vi "Mode Est Acquire Data (TEMP).vi"(7 "Simulation Method":T3(ring), 8 "Simulation?":bool) -> ()   [LabVIEW 2017]
uses:
  <vilib>/Analysis/NI_AALPro.lvlib
  <vilib>/Analysis/NI_AALBase.lvlib
  <vilib>/addons/Control Design/_Time Response Analysis/NI_CD_Time Response.lvlib
  <vilib>/addons/Control Design/_Time Response Analysis/Time Response.llb/Time Response subVI/cd_Linear Simulation (Transfer Function).vi
  <vilib>/addons/Control Design/_Dynamic Analysis/NI_CD_Dynamic Analysis.lvlib
  <vilib>/addons/Control Design/_Dynamic Analysis/Dynamic Analysis.llb/Dynamic Analysis subVI/cd_Damping Ratio and Natural Frequency (Transfer Function).vi
  <vilib>/addons/Control Design/_Model Construction/NI_LinSys_Model Creation.lvlib
  <vilib>/addons/Control Design/_Model Construction/Model Creation.llb/Model Creation SubVI/cd_Create Transfer Function Model.vi
  <vilib>/addons/Control Design/_Model Construction/NI_LinSys_Model Information.lvlib
  <vilib>/addons/Control Design/_Model Construction/Model Information.llb/Model Information SubVIs/cd_Set Names To TF Model.vi
  <vilib>/addons/Control Design/_Utility/NI_CD_Model Viewer.lvlib
  <vilib>/addons/Control Design/_Utility/Model Viewer.llb/Model Viewer SubVI/cd_Draw Transfer Function Equation (TF).vi
  <vilib>/imath/engines/lvmath2/RunTimeEngine/Managers/WorkSpace/UID Generator.vi
  <vilib>/imath/engines/lvmath2/RunTimeEngine/ErrorHandling/NIMS_Error From Error Code.vi
  <vilib>/imath/engines/lvmath2/RunTimeEngine/LocalVariableDefStatement/MC_LocalVariableDefStatement_Display.vi
  <vilib>/imath/engines/lvmath2/RunTimeEngine/RunTimeType/NIMS_RunTimeType_From StrictType (excl LVString).vi
  <vilib>/imath/engines/lvmath2/RunTimeEngine/Managers/SymbolTable/Clear UID.vi
  <vilib>/imath/engines/lvmath2/RunTimeEngine/Managers/SymbolTable/NIMS_WorkSpace.lvlib
  <vilib>/imath/engines/lvmath2/RunTimeEngine/NodeEndStatement/NIMS_NodeEndStatement_Output.vi
  <vilib>/imath/engines/lvmath2/RunTimeEngine/ErrorHandling/NIMS_Finalize Error.vi
  <vilib>/imath/engines/lvmath2/RunTimeEngine/BuiltInFunctions/zpk_to_tf/NIMS_zpk_to_tf.vi
  <vilib>/imath/engines/lvmath/Plug In/_Char/NIMS_CH_String to Character Array.vi
  <vilib>/imath/engines/lvmath2/RunTimeEngine/BuiltInFunctions/fread_csv/NIMS_fread_csv(Str,I32,I32).vi
  <vilib>/imath/engines/lvmath/Plug In/_Char/NIMS_CH_Character RV to String.vi
  sources/support/libs/PMU Buffer/Buffer DATA OUT ordered.ctl
  sources/support/libs/PMU Buffer/PMU data buffer.lvlib
panel:
  in  "Signal Selection":T1(radio)=enum."Analog"
  in  "Sampling Frequency (Hz)":dbl=50.0
  out "Waveform out":waveform(dbl)
  in  "Output":T2
  in  "Acquisition Settings":enum32{"Test", "Simulation", "Options"}(tab)
  in  "Input Poles":cdb[](array[numeric])
  in  "Input Zeros":cdb[](array[numeric])
  in  "CSV File Input (Coefficients)":string
  out "Input Transfer Function":picture
  in  "Input Frequency (Hz)":dbl
  in  "Input Damping Ratio (%)":dbl
  out "Natural Frequencies":dbl[](array[numeric]) format="%.2f"
  out "Damping Ratios (%)":dbl[](array[numeric]) format="%.2f"
  out "Poles":cdb[](array[numeric]) format="%.2f"
  out "Simulation":bool
  # "Create Cluster for simulation inputs"
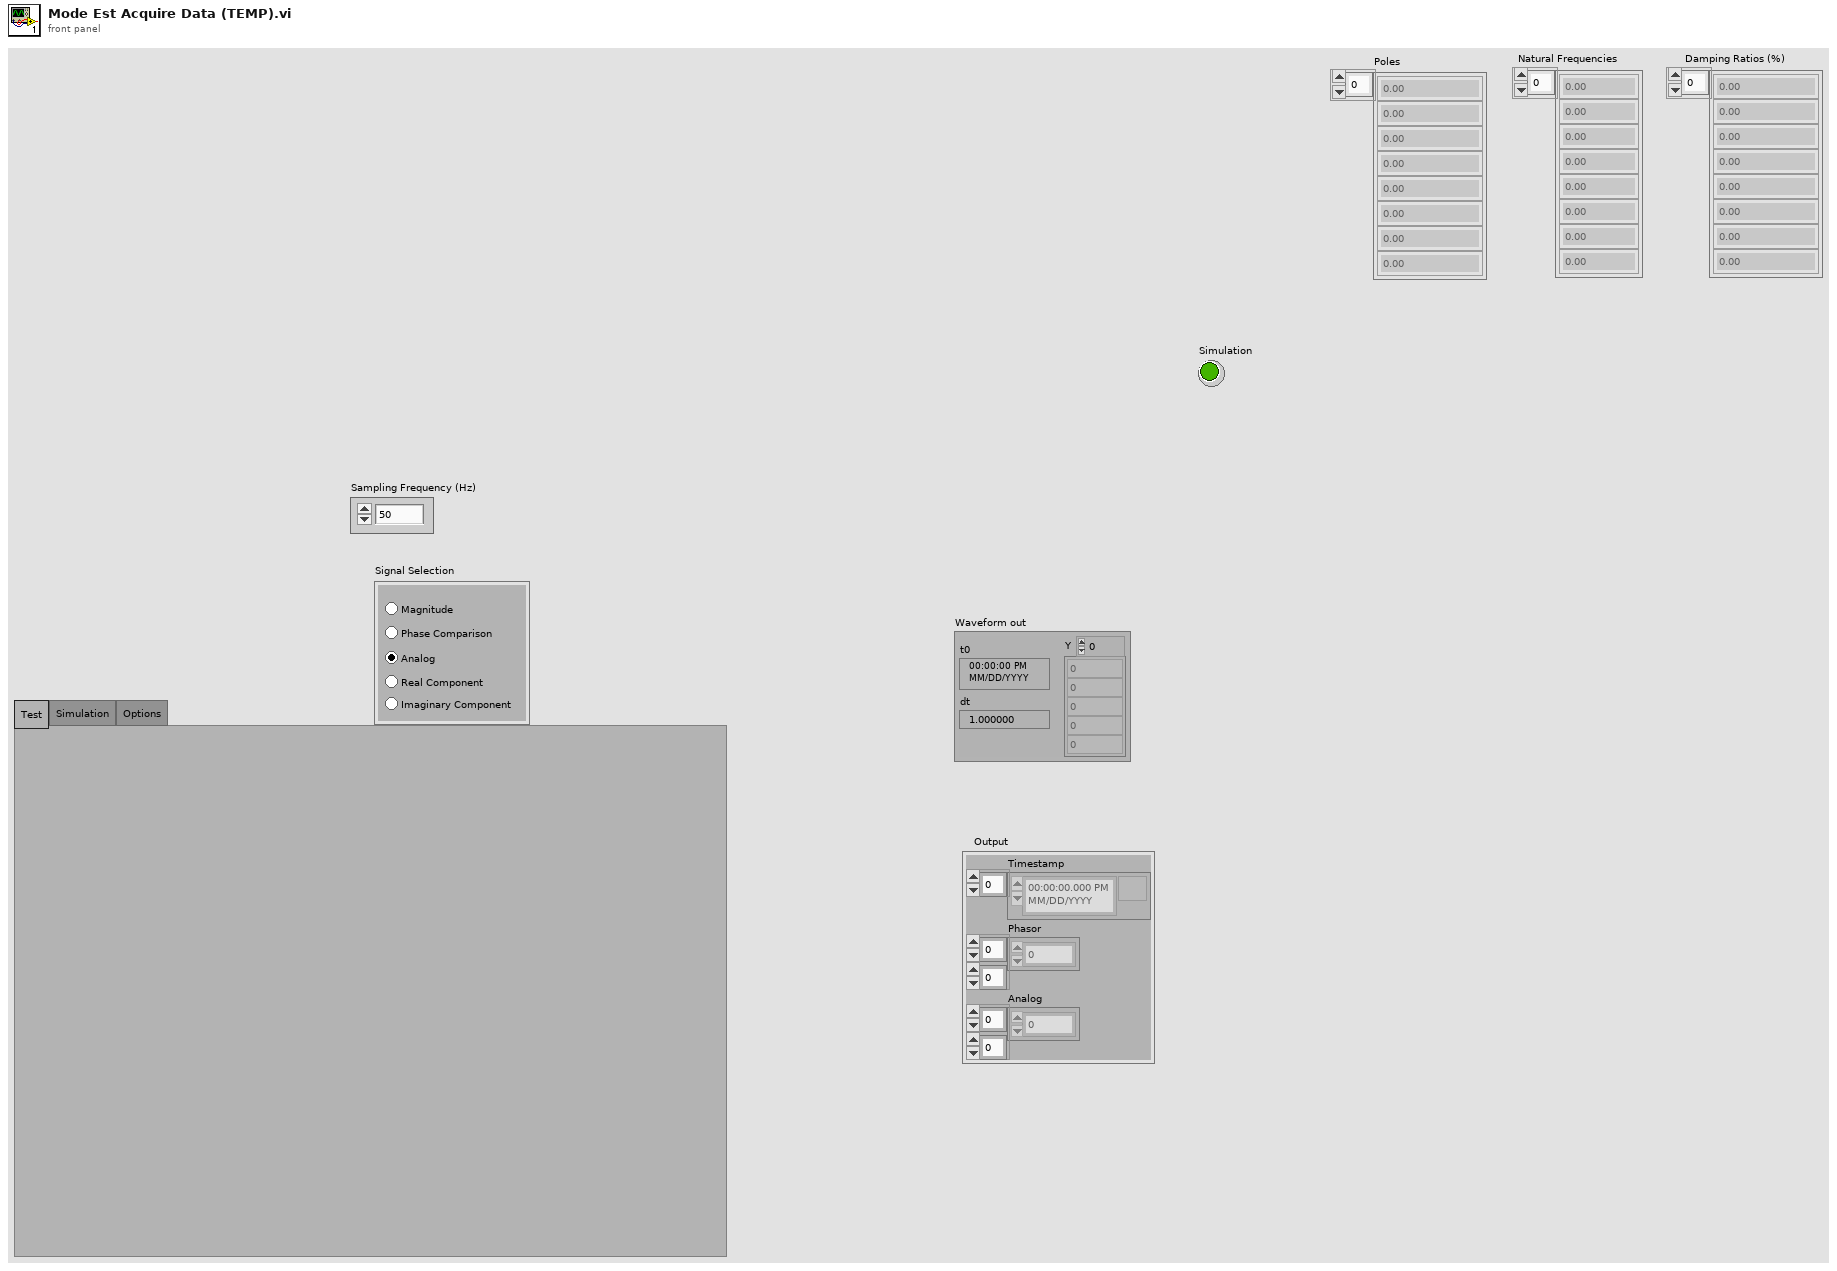
[diagram p1: front panel]
types:
  T1 = enum32{"Mag", "Phase Comparison", "Analog", "Real Component", "Imaginary Component"}
  T2 = typedef "PMU data buffer.lvlib/Buffer DATA OUT ordered.ctl" = cluster{"Timestamp":timestamp[], "Phasor":csg[][], "Analog":sgl[][]}
  T3 = enum16{"Read Coefficients (CSV)", "Use Input Frequency/D.R.", "Use Input Poles/Zeroes"}
  T4 = typedef "NI_LinSys_Model Typedefs.lvlib/CD Transfer Function Model (MIMO).ctl" = cluster{"properties":T5, "transfer function(s)":T6[][]}
  T5 = typedef "NI_LinSys_Model Typedefs.lvlib/CD General Elements.ctl" = cluster{"Model name":string, "Input names":string[], "Output names":string[], "Input Delays":dbl[], "Output Delays":dbl[], "Sampling Time":dbl, "Notes":string}
  T6 = typedef "NI_LinSys_Model Typedefs.lvlib/CD Transfer Function Model (SISO).ctl" = cluster{"Numerator":dbl[], "Denominator":dbl[], "delay":dbl}
  T7 = typedef "NI_LinSys_Data Typedefs.lvlib/CD MIMO Time Response Data.ctl" = cluster{"Time":dbl[], "Outputs Data":dbl[][][], "States Data":dbl[][][], "plot type":T8}
  T8 = typedef "NI_LinSys_Data Typedefs.lvlib/CD Plot Types Enum.ctl" = enum16{"bode-magnitude", "bode-phase", "nichols", "nyquist", "singular values", "step", "impulse", "initial", "simulation", "nyquist with separation"}
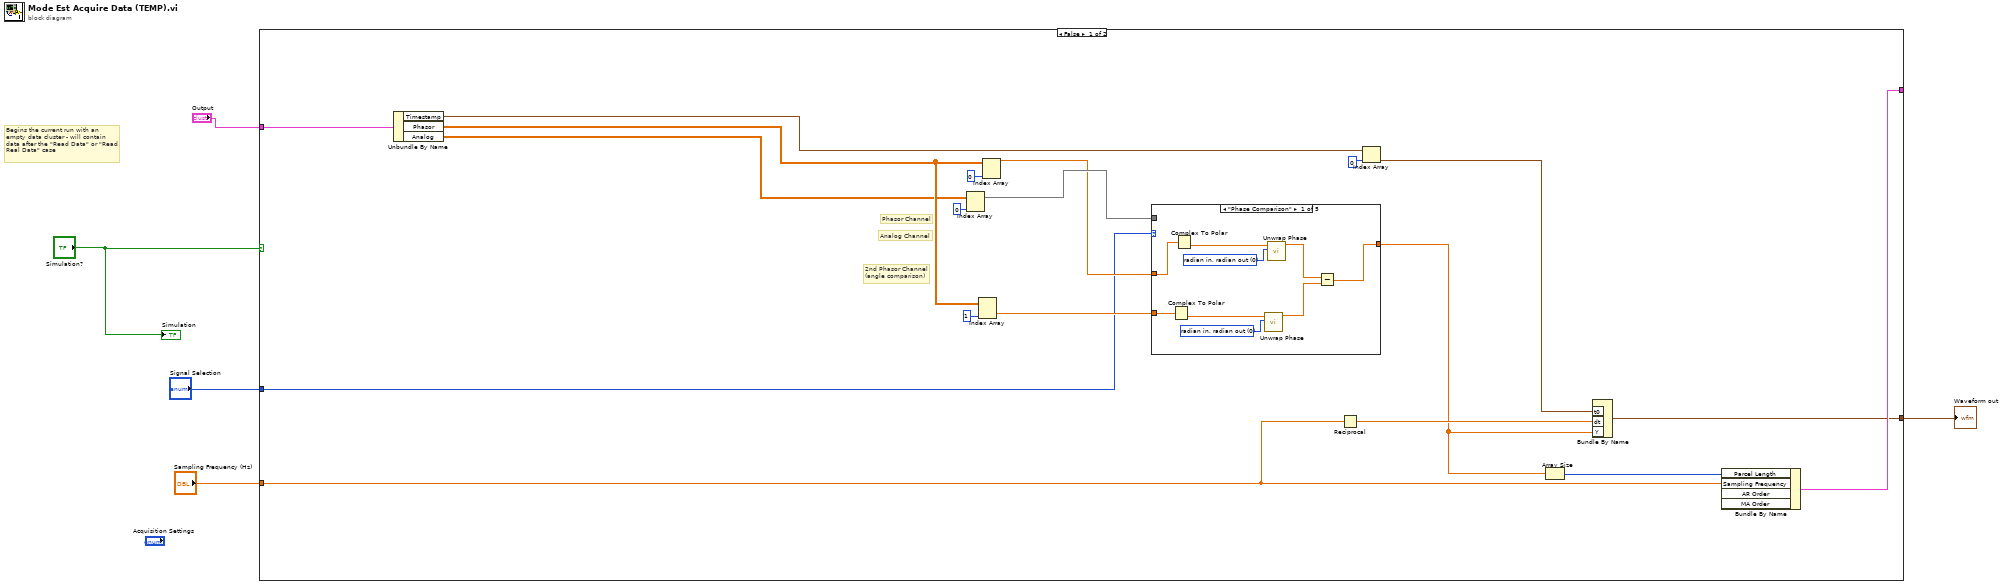
[diagram p0: block diagram]
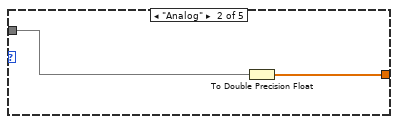
[diagram p2: hidden frame]
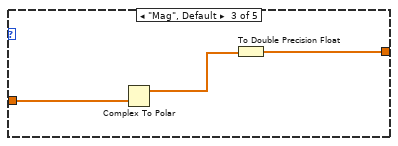
[diagram p3: hidden frame]
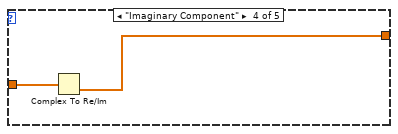
[diagram p4: hidden frame]
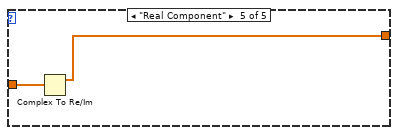
[diagram p5: hidden frame]
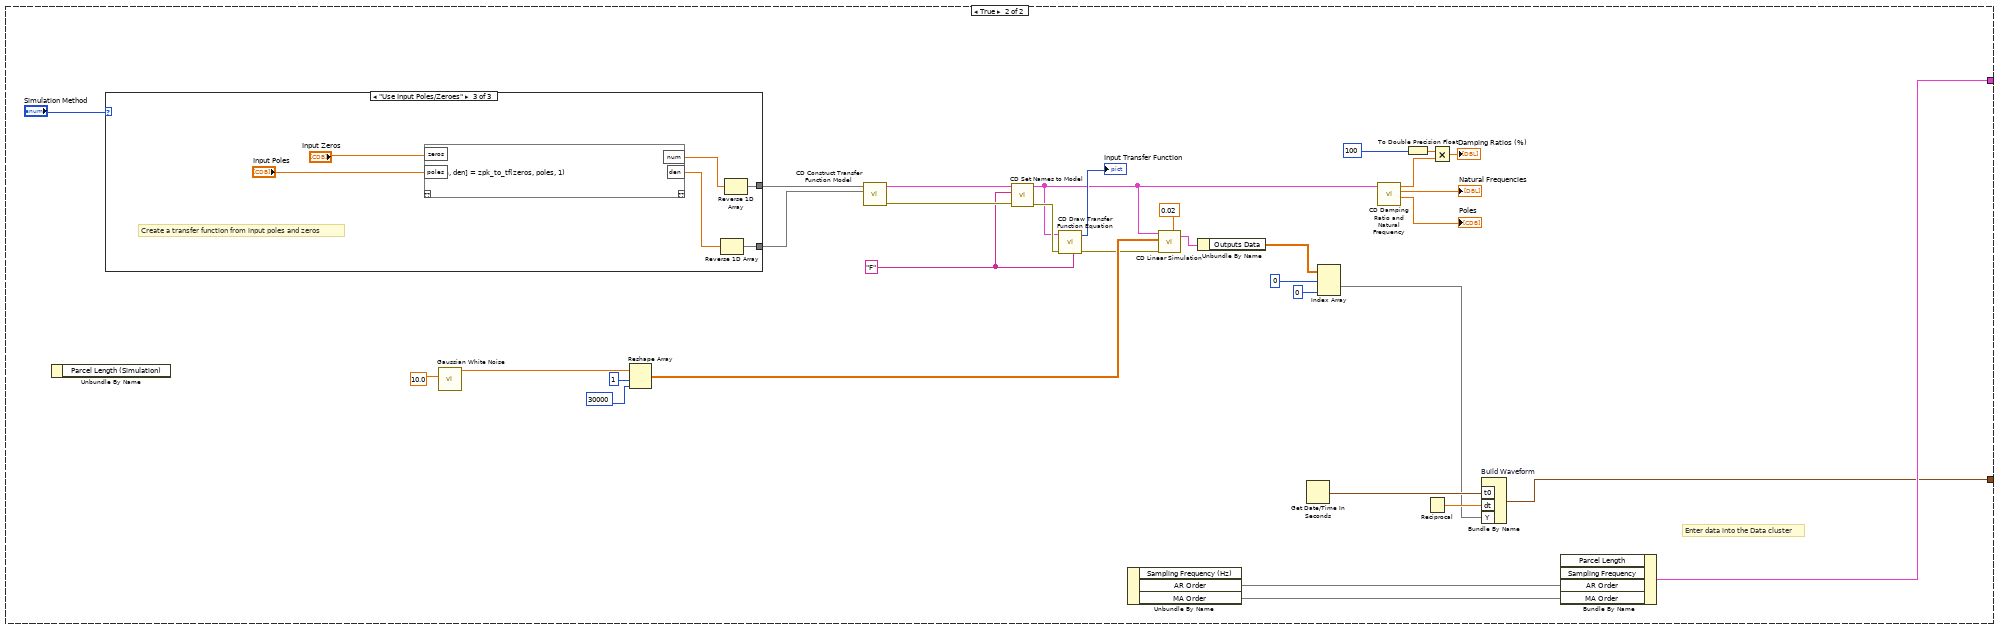
[diagram p6: hidden frame]
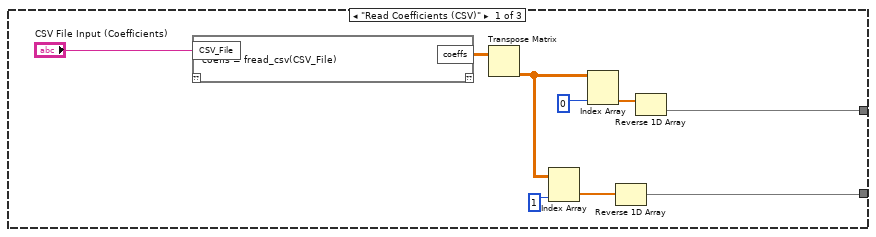
[diagram p7: hidden frame]
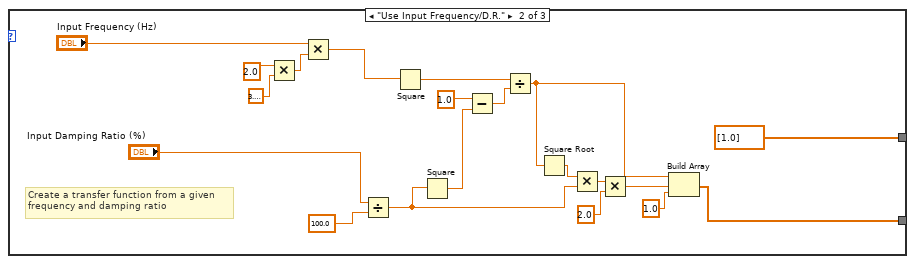
[diagram p8: hidden frame]
diagram:
  # "Begins the current run with an \nempty data cluster - will contain\ndata after the \"Read Data\" or \"Read \nReal Data\" case"
  n1 = case shown="False" "Simulation?" {
    tunnel: [w21 w74] -> _
    tunnel: "Output" -> [w12 _]
    tunnel: [w8 w43] -> w3
    tunnel: "Sampling Frequency (Hz)" -> [w6 _]
    tunnel: "Signal Selection" -> [w7 _]
    frame False {
      # "2nd Phasor Channel\n(angle comparison)"
      # "Analog Channel"
      # "Phasor Channel"
      n2 = Unbundle By Name(w12) -> ("Timestamp"=w11:timestamp[], "Phasor"=w10:csg[][], "Analog"=w9:sgl[][])
      n3 = Index Array "Index Array"(array=w9, index (col)=0 ("disabled index (col)")) -> (element=w19:sgl[])  [unwired: 1 in]
      n4 = Index Array "Index Array"(array=w10, index (col)=1 ("disabled index (col)")) -> (element=w17:csg[])  [unwired: 1 in]
      n5 = Index Array "Index Array"(array=w10, index (col)=0 ("disabled index (col)")) -> (element=w18:csg[])  [unwired: 1 in]
      n6 = case shown="\"Phase Comparison\"" w7 {
        tunnel: [w25 w35 w37 w39 w41] -> w16
        tunnel: w18 -> [w33 _ w38 w40 w42]
        tunnel: w19 -> [_ w34 _ _ _]
        tunnel: w17 -> [w28 _ _ _ _]
        frame "Phase Comparison" {
          w29 = 0 items=["radian in, radian out", "radian in, degree out", "degree in, degree out", "degree in, radian out"] ("phase unit")
          w32 = 0 items=["radian in, radian out", "radian in, degree out", "degree in, degree out", "degree in, radian out"] ("phase unit")
          n7 = Complex To Polar(r * e^(i*theta)=w28) -> (theta=w30:sgl[])  [unwired: 1 out]
          n8 = Complex To Polar(r * e^(i*theta)=w33) -> (theta=w31:sgl[])  [unwired: 1 out]
          n9 = call <vilib>:"Unwrap Phase.vi"("phase unit"=w29, "Phase"=w30) -> ("Unwrapped Phase"=w26:dbl[])  [unwired: 8 in, 1 out]
          n10 = call <vilib>:"Unwrap Phase.vi"("phase unit"=w32, "Phase"=w31) -> ("Unwrapped Phase"=w27:dbl[])  [unwired: 8 in, 1 out]
          n11 = Subtract(x=w27, y=w26) -> (x-y=w25:dbl[])
        }
        frame "Analog" {
          n12 = To Double Precision Float(number=w34) -> (double precision float=w35:dbl[])
        }
        frame "Mag", Default {
          n13 = Complex To Polar(r * e^(i*theta)=w38) -> (r=w36:sgl[])  [unwired: 1 out]
          n14 = To Double Precision Float(number=w36) -> (double precision float=w37:dbl[])
        }
        frame "Imaginary Component" {
          n15 = Complex To Re/Im(x + iy=w40) -> (y=w39:sgl[])  [unwired: 1 out]
        }
        frame "Real Component" {
          n16 = Complex To Re/Im(x + iy=w42) -> (x=w41:sgl[])  [unwired: 1 out]
        }
      }
      n17 = Reciprocal(x=w6) -> (1/x=w24:dbl)
      n18 = Index Array "Index Array"(array=w11, index=0) -> (element=w22:timestamp)
      n19 = Array Size(array=w16) -> (size(s)=w20:i32)
      n20 = Bundle By Name("t0"=w22, "dt"=w24, "Y"=w16) -> (w8:waveform(dbl))  [unwired: 1 in]
      n21 = Bundle By Name("Parcel Length"=w20, "Sampling Frequency"=w6) -> (w21:cluster{})  [unwired: 3 in]
    }
    frame True {
      w53 = "F"
      # "Enter data into the Data cluster"
      n22 = Unbundle By Name() -> ()  [unwired: 1 in, 1 out]
      n23 = case shown="\"Use Input Poles/Zeroes\"" "Simulation Method" {
        tunnel: [w78 dbl[] [1.0] ("Array") w152] -> w51
        tunnel: [w76 w145 w154] -> w50
        frame "Read Coefficients (CSV)" {
          n24 = mathscript code="coeffs = fread_csv(CSV_File)"("CSV_File"="CSV File Input (Coefficients)") -> ("coeffs"=w81:cdb[][])  [unwired: 1 in, 1 out]
          n25 = Transpose Matrix(1:w81) -> (0:w80:cdb[][])
          n26 = Index Array "Index Array"(array=w80, index (col)=1 ("disabled index (col)")) -> (element=w77:cdb[])  [unwired: 1 in]
          n27 = Index Array "Index Array"(array=w80, index (col)=0 ("disabled index (col)")) -> (element=w79:cdb[])  [unwired: 1 in]
          n28 = Reverse 1D Array(array=w77) -> (reversed array=w76:cdb[])
          n29 = Reverse 1D Array(array=w79) -> (reversed array=w78:cdb[])
        }
        frame "Use Input Frequency/D.R." {
          # "Create a transfer function from a given\nfrequency and damping ratio"
          n30 = Multiply(x=2.0 ("y"), y=3.141592653589793) -> (x*y=w147:dbl)
          n31 = Multiply(x="Input Frequency (Hz)", y=w147) -> (x*y=w143:dbl)
          n32 = Divide(x="Input Damping Ratio (%)", y=100.0) -> (x/y=w133:dbl)
          n33 = Square(x=w143) -> (x^2=w142:dbl)
          n34 = Square(x=w133) -> (x^2=w136:dbl)
          n35 = Subtract(x=1.0 ("standard deviation"), y=w136) -> (x-y=w135:dbl)
          n36 = Divide(x=w142, y=w135) -> (x/y=w134:dbl)
          n37 = Square Root(x=w134) -> (sqrt(x)=w138:dbl)
          n38 = Multiply(x=w138, y=w133) -> (x*y=w139:dbl)
          n39 = Multiply(x=w139, y=2.0) -> (x*y=w141:dbl)
          n40 = Build Array(w134, w141, 1.0 ("standard deviation")) -> (w145:dbl[])
        }
        frame "Use Input Poles/Zeroes" {
          # "Create a transfer function from input poles and zeros"
          n41 = mathscript code="[num, den] = zpk_to_tf(zeros, poles, 1)"("zeros"="Input Zeros", "poles"="Input Poles") -> ("num"=w153:dbl[], "den"=w155:dbl[])  [unwired: 1 in, 1 out]
          n42 = Reverse 1D Array(array=w155) -> (reversed array=w154:dbl[])
          n43 = Reverse 1D Array(array=w153) -> (reversed array=w152:dbl[])
        }
      }
      n44 = call <vilib>:"Gaussian White Noise.vi"("standard deviation"=10.0) -> ("Gaussian noise pattern"=w71:dbl[])  [unwired: 9 in, 1 out]
      n45 = Reshape Array "Reshape Array"(w71, 1 ("dimension size"), 30000 ("dimension size")) -> (w70:dbl[][])
      n46 = call-poly <vilib>:"CD Construct Transfer Function Model.vi"("Denominator"=w50, "Numerator"=w51) -> ("error out"=w54:errorcluster, "Transfer Function Model"=w56:T4)  [unwired: 8 in]
      n47 = call-poly <vilib>:"CD Set Names to Model.vi"("Model Name"=w53, "Transfer Function Model In"=w56, "error in (no error)"=w54) -> ("Model Out"=w44:T4, "error out"=w55:errorcluster)  [unwired: 11 in]
      n48 = call-poly <vilib>:"CD Draw Transfer Function Equation.vi"("Function Name (empty)"=w53, "error in (no error)"=w55, "Transfer Function Model"=w44) -> ("error out"=w52:errorcluster, "Equation"=→"Input Transfer Function":picture)  [unwired: 6 in, 1 out]
      n49 = Unbundle By Name() -> ("AR Order"=w47, "MA Order"=w46)  [unwired: 1 in, 1 out]
      n50 = call-poly <vilib>:"CD Linear Simulation.vi"("Delta t"=0.02, "error in (no error)"=w52, "Inputs"=w70, "Transfer Function Model"=w44) -> ("Simulation Data"=w69:T7)  [unwired: 5 in, 2 out]
      n51 = Unbundle By Name(w69) -> ("Outputs Data"=w66:dbl[][][])
      n52 = Get Date/Time In Seconds() -> (seconds since 1Jan1904=w73:timestamp)
      n53 = Index Array "Index Array"(array=w66, index (dim 0)=0 ("index"), index (dim 2)=0 ("length")) -> (element=w45:dbl[])  [unwired: 1 in]
      n54 = call-poly <vilib>:"CD Damping Ratio and Natural Frequency.vi"("Transfer Function Model"=w44) -> ("Poles"=→"Poles":cdb[], "Natural Frequencies"=→"Natural Frequencies":dbl[], "Damping Ratios"=w61:dbl[])  [unwired: 7 in, 1 out]
      n55 = To Double Precision Float(number=100 ("length")) -> (double precision float=w58:dbl)
      n56 = Reciprocal() -> (1/x=w75:dbl)  [unwired: 1 in]
      n57 = Multiply(x=w58, y=w61) -> (x*y=→"Damping Ratios (%)":dbl[])
      n58 = Bundle By Name "Build Waveform"("t0"=w73, "dt"=w75, "Y"=w45) -> (w43:waveform(dbl))  [unwired: 1 in]
      n59 = Bundle By Name("AR Order"=w47, "MA Order"=w46) -> (w74:cluster{})  [unwired: 3 in]
    }
  }
  "Waveform out" <- w3
  "Simulation" <- "Simulation?"
